vi "Save Configuration.vi"(8 "error in (no error)":errorcluster, 10 "Save As?":bool, 11 "Cfg Grandmaster in":refnum<class "Cfg Grandmaster.lvclass">) -> (0 "error out":errorcluster, 3 "Cfg Grandmaster out":refnum<class "Cfg Grandmaster.lvclass">)   [LabVIEW 2018, in "Configuration Grandmaster.lvlib" / "Cfg Grandmaster.lvclass"]
uses:
  Cfg Grandmaster.lvclass
  Cfg Grandmaster.lvclass/Cfg Grandmaster.ctl
  Class Chassis BOM/Chassis BOM.lvclass/Chassis BOM.ctl
  Class Chassis BOM/Write CfgFile.vi
  Class Chassis BOM/Read Chassis Alias.vi
  Class Chassis Cfg/ChassisCfg.lvclass
  Class Chassis BOM/Chassis BOM.lvclass
  <vilib>/NI/GXML/GXML.lvlib
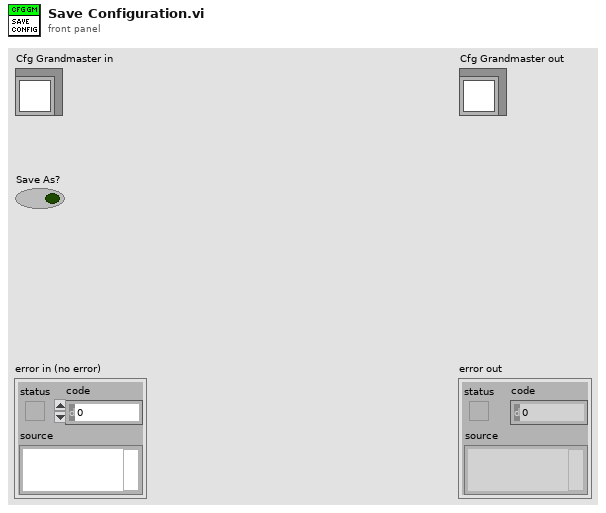
[diagram p1: front panel]
types:
  T1 = typedef "ge_Cfg wChassis.ctl" = cluster{"Chassis BOM":refnum<class "Chassis BOM.lvclass">, "Chassis Cfg":refnum<class "ChassisCfg.lvclass">, "Chassis Tasks":refnum<class "Chassis Tasks.lvclass">, "HW Error":bool, "Unsvd Chgs?":bool}
  T2 = enum16{"Left Button", "Center Button", "Right Button", "Window Close"}
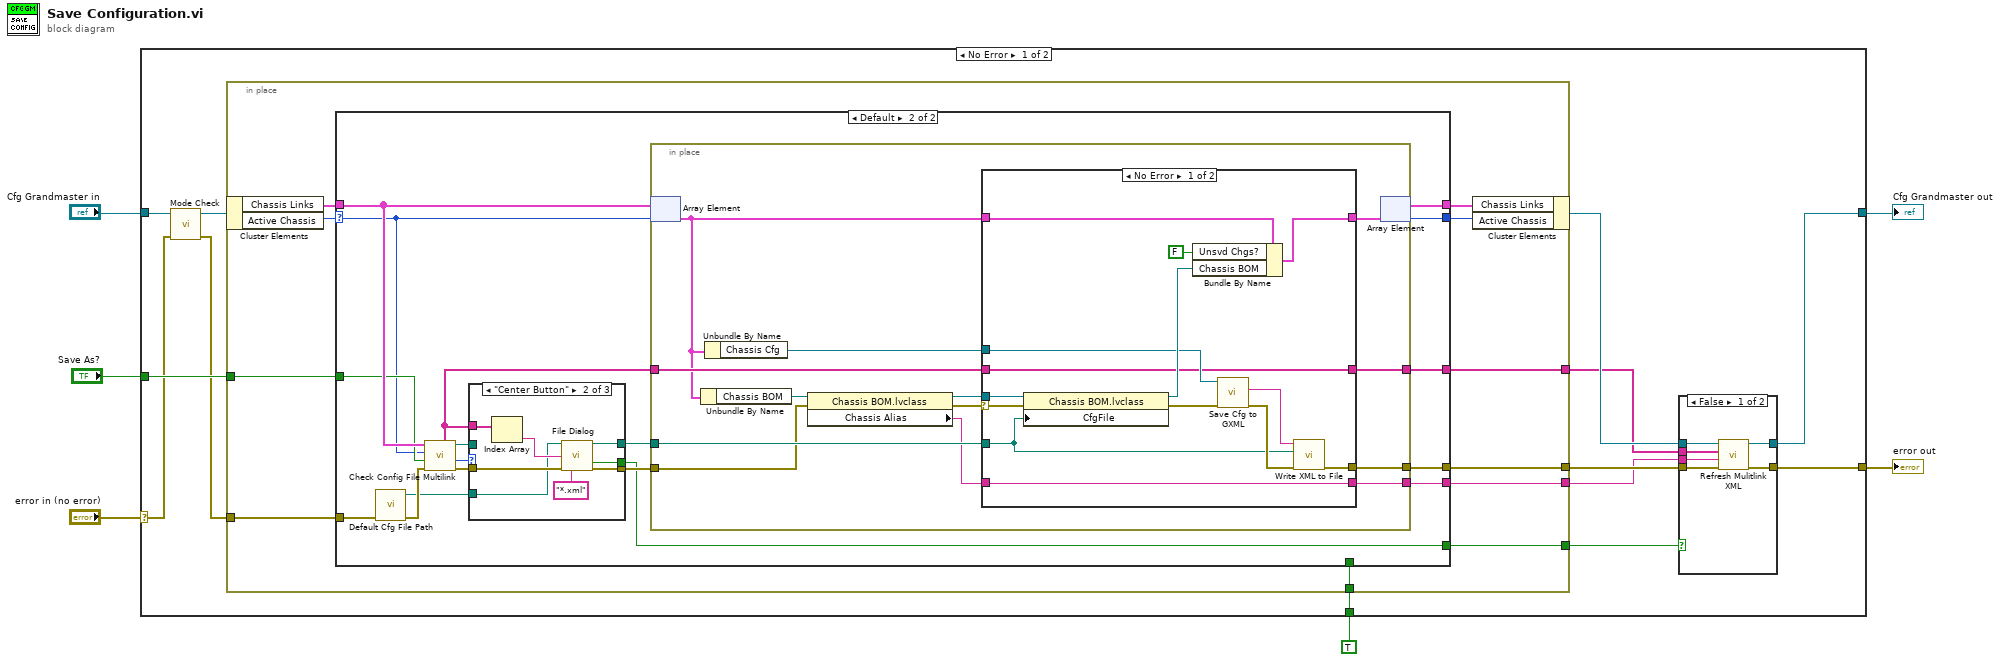
[diagram p0: block diagram]
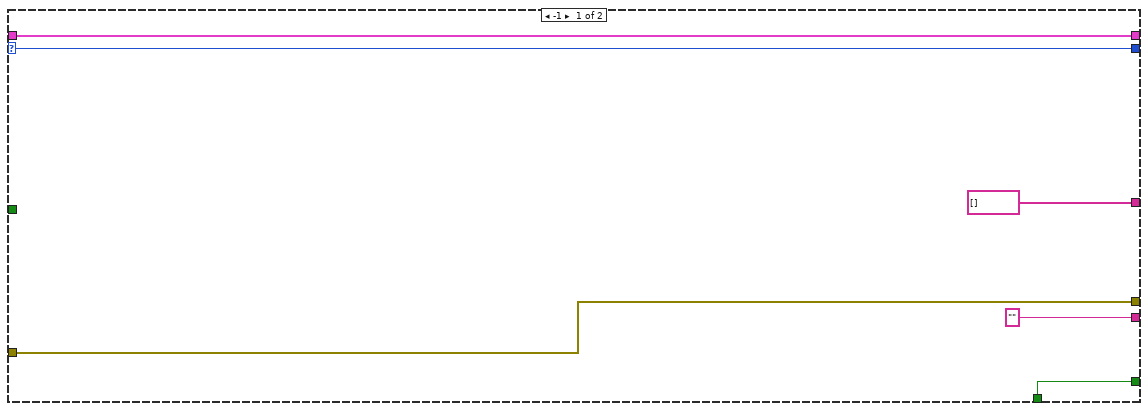
[diagram p3: hidden frame]
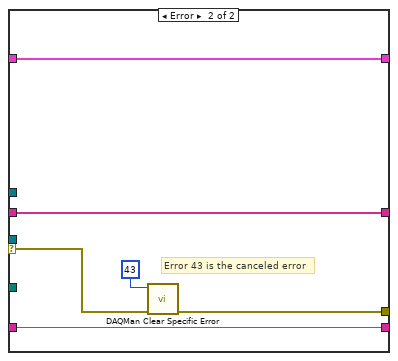
[diagram p4: hidden frame]
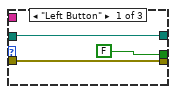
[diagram p5: hidden frame]
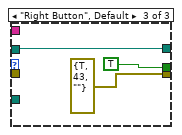
[diagram p6: hidden frame]
diagram:
  n1 = case shown="No Error" "error in (no error)" {
    selector: "error in (no error)" -> [w15 w111]
    tunnel: [w8 w111] -> w5
    tunnel: [w9 w110] -> w3
    tunnel: "Cfg Grandmaster in" -> [w17 w110]
    tunnel: "Save As?" -> [w19 _]
    tunnel: TRUE ("cancelled") -> [w18 _]
    frame No Error {
      n2 = call "Mode Check.vi"("error in (no error)"=w15, "Cfg Grandmaster in"=w17) -> ("error out"=w14:errorcluster, "Cfg Grandmaster out"=w16:refnum<class "Cfg Grandmaster.lvclass">)  [unwired: 8 in]
      n3 = in-place {
        in-place-border: w19 -> [w37]
        in-place-border: w14 -> [w33]
        in-place-border: [w32] -> w12
        in-place-border: [w31] -> w7
        in-place-border: w18 -> [w30]
        in-place-border: [w29] -> w11
        in-place-border: [w28] -> w10
        n4 = in-place-cluster #1(w16) -> ("Chassis Links"=w38:T1[], "Active Chassis"=w35:i32)
        n5 = case shown="Default" w35 {
          selector: w35 -> [w42 w47]
          tunnel: [w43 w62] -> w32
          tunnel: [w41 w60] -> w31
          tunnel: w38 -> [w44 w55]
          tunnel: w33 -> [w43 w52]
          tunnel: [w44 w54] -> w36
          tunnel: w37 -> [_ w49]
          tunnel: [w42 w48] -> w34
          tunnel: w30 -> [w41 _]
          tunnel: [string[] [] ("Referencing Chassis") w46] -> w29
          tunnel: ["" ("Chassis Name") w45] -> w28
          frame -1 {
          }
          frame Default {
            n6 = call "Default Cfg File Path.vi"("error in (no error)"=w52) -> ("error out"=w51:errorcluster, "Default Path"=w50:path)  [unwired: 9 in]
            n7 = call "Check Config File Multilink.vi"("error in (no error)"=w51, "Save As?"=w49, "Index"=w47, "cDAQ Configs"=w55) -> ("error out"=w53:errorcluster, "Which Button?"=w57:T2, "CfgFile Path"=w58:path, "Referencing Chassis"=w56:string[])  [unwired: 4 in]
            n8 = case shown="\"Center Button\"" w57 {
              tunnel: [w97 w106 w109] -> w59
              tunnel: [w98 w104 errorcluster {"status"=TRUE, "code"=43, "source"=""} ("error out")] -> w61
              tunnel: w58 -> [w97 _ w109]
              tunnel: w53 -> [w98 w105 _]
              tunnel: [FALSE ("cancelled") w103 TRUE ("cancelled")] -> w60
              tunnel: w56 -> [_ w101 _]
              tunnel: w50 -> [_ w99 _]
              frame "Left Button" {
              }
              frame "Center Button" {
                n9 = Index Array(array=w101) -> (element=w100:string)  [unwired: 1 in]
                n10 = call "File Dialog"("start path"=w99, "default name"=w100, "error in"=w105, "pattern (all files)"="*.xml") -> ("selected path"=w106:path, "cancelled"=w103:bool, "error out"=w104:errorcluster)  [unwired: 8 in, 1 out]
              }
              frame "Right Button", Default {
              }
            }
            n11 = in-place {
              in-place-border: [w75] -> w62
              in-place-border: w61 -> [w71]
              in-place-border: w59 -> [w74]
              in-place-border: w56 -> [w69]
              in-place-border: [w64] -> w46
              in-place-border: [w63] -> w45
              n12 = in-place-array #2(w55, w47) -> (w66:T1)
              n13 = Unbundle By Name(w66) -> ("Chassis BOM"=w72:refnum<class "Chassis BOM.lvclass">)
              n14 = Unbundle By Name(w66) -> ("Chassis Cfg"=w65:refnum<class "ChassisCfg.lvclass">)
              n15 = property class="Chassis BOM.lvclass"(reference=w72, error in=w71) -> (reference out=w67:refnum<class "Chassis BOM.lvclass">, error out=w70:errorcluster, "Chassis Alias"=w68:string)
              n16 = case shown="No Error" w70 {
                selector: w70 -> [w82 w94]
                tunnel: [w78 w93] -> w75
                tunnel: w74 -> [w84 _]
                tunnel: w66 -> [w89 w95]
                tunnel: [w85 w95] -> w73
                tunnel: w69 -> [w77 w90]
                tunnel: w68 -> [w76 w91]
                tunnel: w67 -> [w83 _]
                tunnel: w65 -> [w79 _]
                tunnel: [w77 w90] -> w64
                tunnel: [w76 w91] -> w63
                frame No Error {
                  n17 = property class="Chassis BOM.lvclass"(reference=w83, error in=w82, "CfgFile"=w84) -> (reference out=w80:refnum<class "Chassis BOM.lvclass">, error out=w81:errorcluster)
                  n18 = Bundle By Name(cluster=w89, "Unsvd Chgs?"=FALSE, "Chassis BOM"=w80) -> (w85:T1)
                  n19 = call "Save Cfg to GXML.vi"("error in"=w81, "Chassis Cfg"=w79) -> ("error out"=w87:errorcluster, "GXML String"=w86:string)  [unwired: 8 in]
                  n20 = call <vilib>:"Write XML to File.vi"("error in"=w87, "XML File Path"=w84, "XML Input"=w86) -> ("error out"=w78:errorcluster)  [unwired: 8 in]
                }
                frame Error {
                  # "Error 43 is the canceled error"
                  n21 = call "DAQMan Clear Specific Error.vi"("error in"=w94, "code"=43 ("y")) -> ("error out"=w93:errorcluster)  [unwired: 9 in]
                }
              }
              n22 = in-place-array #2(w73) -> (w54:T1[], w48:i32)
            }
          }
        }
        n23 = in-place-cluster #1("Chassis Links"=w36, "Active Chassis"=w34) -> (w13:refnum<class "Cfg Grandmaster.lvclass">)
      }
      n24 = case shown="False" w7 {
        tunnel: w13 -> [w25 w27]
        tunnel: w12 -> [w24 w26]
        tunnel: w11 -> [w23 _]
        tunnel: w10 -> [w22 _]
        tunnel: [w21 w27] -> w9
        tunnel: [w20 w26] -> w8
        frame False {
          n25 = call "Refresh Mulitlink XML.vi"("error in"=w24, "Chassis Name"=w22, "Referencing Chassis"=w23, "Cfg GM"=w25) -> ("error out"=w20:errorcluster, "Cfg GM"=w21:refnum<class "Cfg Grandmaster.lvclass">)  [unwired: 6 in]
        }
        frame True {
        }
      }
    }
    frame Error {
    }
  }
  "error out" <- w5
  "Cfg Grandmaster out" <- w3
